vi "Query Register Values.vi"(8 "error in (no error)":errorcluster, 9 "Query Register Value (0:Service request Enable)":u16(ring) items=["Service request Enable", "Standard Event Status Enable", "Standard Event Status Register", "Status Byte"], 11 "VISA resource name":refnum<visa-resource-name>) -> (0 "error out":errorcluster, 2 "Register Value":i16, 3 "VISA resource name out":refnum<visa-resource-name>)   [LabVIEW 2018, in "LTB-1.lvlib" / "3150.lvlib"]
doc: "Queries the Register values for different commands."
uses:
  3150.lvlib
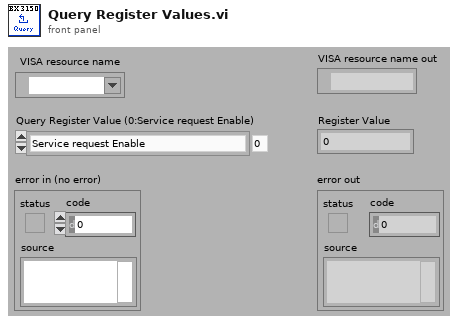
[diagram p1: front panel]
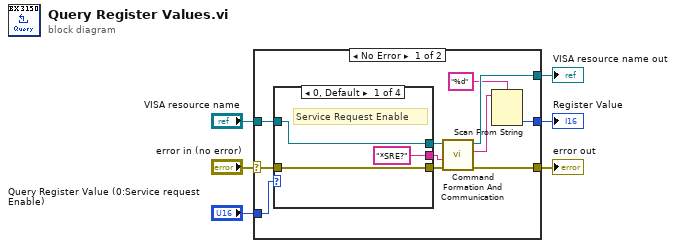
[diagram p0: block diagram]
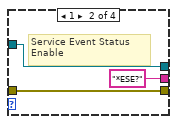
[diagram p2: hidden frame]
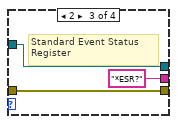
[diagram p3: hidden frame]
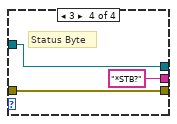
[diagram p4: hidden frame]
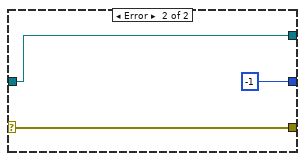
[diagram p5: hidden frame]
diagram:
  n1 = case shown="No Error" "error in (no error)" {
    selector: "error in (no error)" -> [w16 w32]
    tunnel: [w7 -1] -> w6
    tunnel: "VISA resource name" -> [w17 w31]
    tunnel: [w9 w32] -> w1
    tunnel: [w12 w31] -> w4
    tunnel: "Query Register Value (0:Service request Enable)" -> [w15 _]
    frame No Error {
      n2 = case shown="0, Default" w15 {
        tunnel: w17 -> [w20 w22 w25 w28]
        tunnel: w16 -> [w19 w21 w24 w27]
        tunnel: [w20 w22 w25 w28] -> w14
        tunnel: [w19 w21 w24 w27] -> w13
        tunnel: ["*SRE?" ("Command") "*ESE?" ("Command") "*ESR?" ("Command") "*STB?" ("Command")] -> w10
        frame 0, Default {
          # "Service Request Enable"
        }
        frame 1 {
          # "Service Event Status \nEnable"
        }
        frame 2 {
          # "Standard Event Status \nRegister"
        }
        frame 3 {
          # "Status Byte"
        }
      }
      n3 = call "Command Formation And Communication.vi"("error in (no error)"=w13, "Command"=w10, "VISA resource name"=w14) -> ("error out"=w9:errorcluster, "Response"=w11:string, "VISA resource name out"=w12:refnum<visa-resource-name>)  [unwired: 1 in, 5 out]
      n4 = Scan From String(format string="%d", input string=w11) -> (output 1=w7:i32)  [unwired: 2 in, 4 out]
    }
    frame Error {
    }
  }
  "Register Value" <- w6
  "VISA resource name out" <- w4
  "error out" <- w1
